vi "ReturnFrame.vi"(2 "Data Values In":u16[](graph) caption="Data Values", 3 "curr_nob":u32=1, 4 "curr_nos":u32=1, 5 "Drv":u32=1) -> (0 "Data Values Out":u16[](graph) caption="Data Values")   [LabVIEW 2015]
uses:
  ESLSCDLL.dll
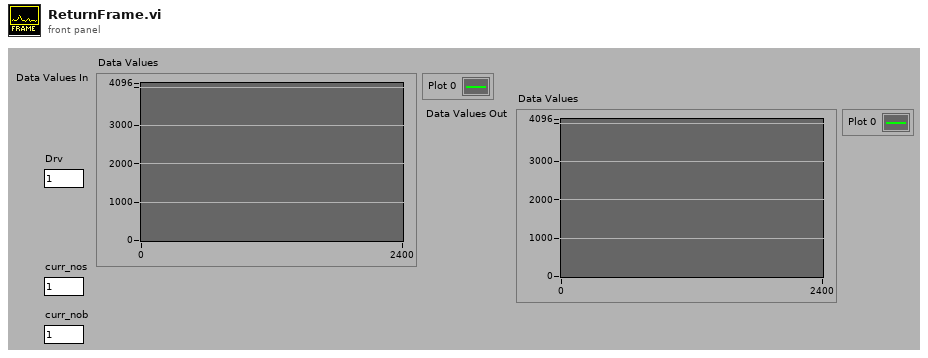
[diagram p1: front panel]
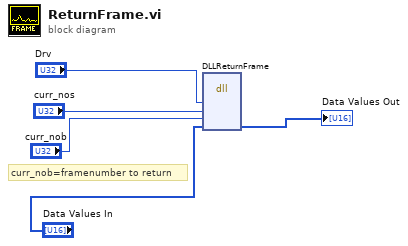
[diagram p0: block diagram]
diagram:
  # "curr_nob=framenumber to return"
  n1 = dll-call lib="C:/ENTW/PCIE/64bit/lv64/lv64_labview2015/board.vis/ESLSCDLL.dll" fn="DLLReturnFrame" ("lwlscdll.dll:DLLReadFFLoop")("drv"="Drv", "curr_nos"="curr_nos", "curr_nob"="curr_nob", "dioden"="Data Values In") -> ("dioden"=→"Data Values Out":u16[])  [unwired: 7 in, 2 out]
